vi "New Container.vi"(8 "error in (no error)":errorcluster, 11 "Engine in":refnum<class "Engine.lvclass">) -> (0 "error out":errorcluster, 2 "New PropertyObject":refnum<class "PropertyObject.lvclass">, 3 "Engine out":refnum<class "Engine.lvclass">)   [LabVIEW 2020, in "TSnax.lvlib" / "Engine.lvclass"]
uses:
  Engine.lvclass
  Engine.lvclass/Engine.ctl
  VariableContainer Type.ctl
  PropertyObject/PropertyObject.lvclass
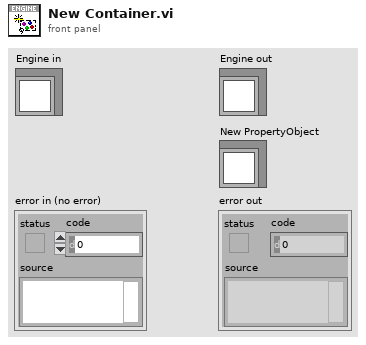
[diagram p1: front panel]
types:
  T1 = typedef "TSnax.lvlib/Engine.lvclass/VariableContainer Type.ctl" = enum16{"StationGlobals", "TemporaryGlobals", "NewPropertyObject", "SubProperty"}
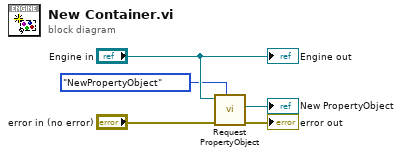
[diagram p0: block diagram]
diagram:
  n1 = call "Request PropertyObject.vi"("Type"=VariableContainer_Type."NewPropertyObject", "error in (no error)"="error in (no error)", "Engine in"="Engine in") -> ("error out"=→"error out":errorcluster, "PropertyObject"=→"New PropertyObject":refnum<class "PropertyObject.lvclass">)  [unwired: 7 in]
  "Engine out" <- "Engine in"
